vi "Catch Nested Value Update.vi"(8 "error in (no error)":errorcluster, 10 "Nested Value Update Msg":refnum<class "Nested Value Update Msg.lvclass">, 11 "IViewModel In":refnum<class "IViewModel.lvclass">) -> (0 "error out":errorcluster, 3 "IViewModel Out":refnum<class "IViewModel.lvclass">)   [LabVIEW 2015, in "IViewModel.lvlib" / "IViewModel.lvclass"]
doc: "<License>\nCopyright © 2017 Composed Systems, LLC | All rights reserved\nwww.composed.io\n\nAuthor: Ethan Stern <ethan.stern@composed.io>\n\nThis software is provided \"AS IS\" WITHOUT WARRANTIES, either express or implied, AND IS FOR EDUCATIONAL PURPOSES ONLY.\n</License>"
uses:
  IViewModel.lvclass
  IViewable/IViewable Messages/Catch Nested Value Change Msg/Nested Value Update Msg.lvclass
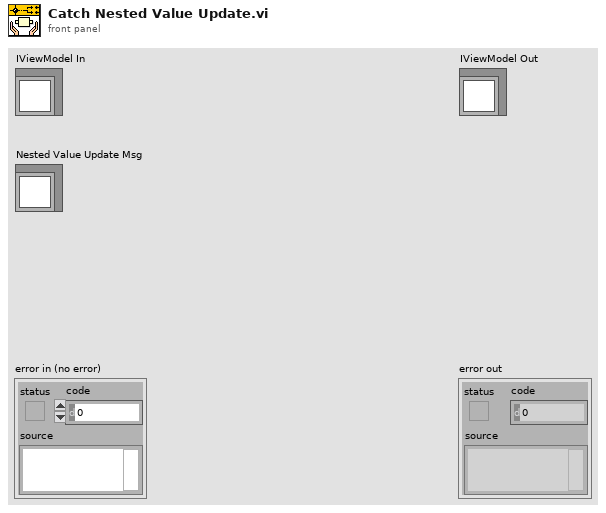
[diagram p1: front panel]
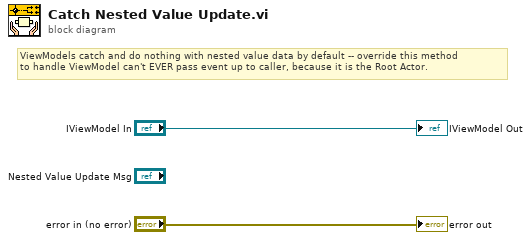
[diagram p0: block diagram]
diagram:
  # "ViewModels catch and do nothing with nested value data by default -- override this method\nto handle ViewModel can't EVER pass event up to caller, because it is the Root Actor."
  "error out" <- "error in (no error)"
  "IViewModel Out" <- "IViewModel In"
